vi "Test Initiate.vi"(0 "Template Tx Test in":refnum<class "niDTS WLAN Tx Test.lvclass">, 11 "error in (no error)":errorcluster) -> (4 "Template Tx Test out":refnum<class "niDTS WLAN Tx Test.lvclass">, 15 "error out":errorcluster)   [LabVIEW 2015, in "niDTS WLAN.lvlib" / "niDTS WLAN Tx Test.lvclass"]
uses:
  niDTS WLAN Tx Test.lvclass
  Instrument/INSTR TX/niDTS WLAN INSTR TX.lvclass
  Framework/Dut/Objects/BASE_class/niDTS Dut.lvclass
  Dut/Objects/BASE_class/niDTS WLAN Dut.lvclass
  niDTS WLAN.lvlib
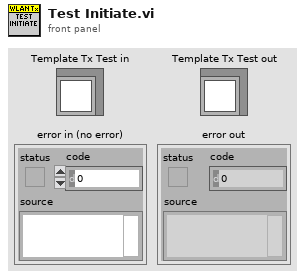
[diagram p1: front panel]
types:
  T1 = typedef "niDTS Framework.lvlib/niDTS Dut INC Handle.ctl" = refnum<data-value>
  T2 = typedef "niDTS WLAN.lvlib/niDTS WLAN Dut INC Handle.ctl" = refnum<data-value>
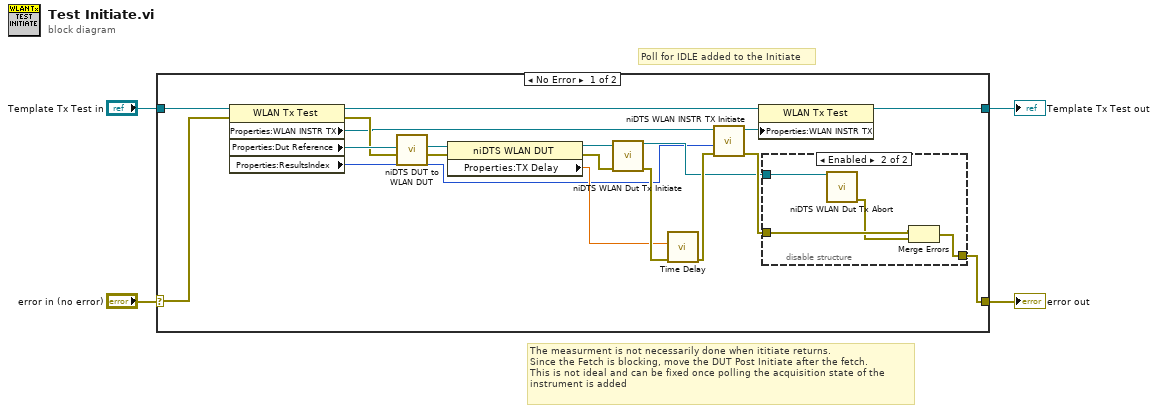
[diagram p0: block diagram]
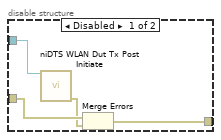
[diagram p2: hidden frame]
diagram:
  # "Poll for IDLE added to the Initiate"
  # "The measurment is not necessarily done when ititiate returns.\nSince the Fetch is blocking, move the DUT Post Initiate after the fetch.\nThis is not ideal and can be fixed once polling the acquisition state of the\ninstrument is added"
  n1 = case shown="No Error" "error in (no error)" {
    selector: "error in (no error)" -> [w23 w33]
    tunnel: [w7 w33] -> w3
    tunnel: [w10 w32] -> w1
    tunnel: "Template Tx Test in" -> [w22 w32]
    frame No Error {
      n2 = property class="WLAN Tx Test"(reference=w22, error in=w23) -> (reference out=w12:refnum<class "niDTS WLAN Tx Test.lvclass">, error out=w20:errorcluster, "Properties:WLAN INSTR TX"=w6:refnum<class "niDTS WLAN INSTR TX.lvclass">, "Properties:Dut Reference"=w21:T1, "Properties:ResultsIndex"=w5:u8)
      n3 = call "niDTS DUT to WLAN DUT.vi"("error in"=w20, "Dut Handle"=w21) -> ("error out"=w18:errorcluster, "WLAN Dut Handle"=w19:T2)  [unwired: 8 in]
      n4 = property class="niDTS WLAN DUT"(reference=w19, error in=w18) -> (reference out=w17:T2, error out=w16:errorcluster, "Properties:TX Delay"=w14:dbl)
      n5 = call "niDTS WLAN Dut Tx Initiate.vi"("Dut Handle in"=w17, "error in (no error)"=w16) -> ("Dut Handle out"=w8:T1, "error out"=w15:errorcluster)  [unwired: 12 in]
      n6 = call "Time Delay"("error in (no error)"=w15, "Delay Time (s)"=w14) -> ("error out"=w13:errorcluster)  [unwired: 9 in]
      n7 = call-dynamic "niDTS WLAN INSTR TX Initiate.vi"("error in (no error)"=w13, "Result Instance"=w5, "niDTS WLAN INSTR TX in"=w6) -> ("error out"=w9:errorcluster, "niDTS WLAN INSTR TX out"=w11:refnum<class "niDTS WLAN INSTR TX.lvclass">)  [unwired: 7 in]
      n8 = property class="WLAN Tx Test"(reference=w12, "Properties:WLAN INSTR TX"=w11) -> (reference out=w10:refnum<class "niDTS WLAN Tx Test.lvclass">)  [unwired: 1 in, 1 out]
      n9 = disable-structure shown="Enabled" {
        disable-tunnel: w9 -> [w26 w30]
        disable-tunnel: w8 -> [w27 w31]
        disable-tunnel: [w24 w28] -> w7
        frame Disabled {
          n10 = call "niDTS WLAN Dut Tx Post Initiate.vi"("Dut Handle in"=w27) -> ("error out"=w25:errorcluster)  [unwired: 13 in, 1 out]
          n11 = Merge Errors(w26, w25) -> (w24:errorcluster)
        }
        frame Enabled {
          n12 = call "niDTS WLAN Dut Tx Abort.vi"("WLAN Dut Handle in"=w31) -> ("error out"=w29:errorcluster)  [unwired: 13 in, 1 out]
          n13 = Merge Errors(w30, w29) -> (w28:errorcluster)
        }
      }
    }
    frame Error {
    }
  }
  "error out" <- w3
  "Template Tx Test out" <- w1
